vi "niDTS WLAN INSTR TX Configure Trigger.vi"(8 "error in (no error)":errorcluster, 11 "niDTS WLAN INSTR TX in":refnum<class "niDTS WLAN INSTR TX.lvclass">) -> (0 "error out":errorcluster, 3 "niDTS WLAN INSTR TX out":refnum<class "niDTS WLAN INSTR TX.lvclass">)   [LabVIEW 2015, in "niDTS WLAN.lvlib" / "niDTS WLAN INSTR TX.lvclass"]
doc: "Sets:\n\n* TriggerThreshold\n* Trigger Source\n* MinQuietTimeDuration\n* TriggerTimeout"
uses:
  niDTS WLAN INSTR TX.lvclass
  niDTS WLAN INSTR TX.lvclass/niDTS WLAN INSTR TX.ctl
  RiviInstDriver/niRfsaWlan/Objects/niRfsaWlan.lvclass
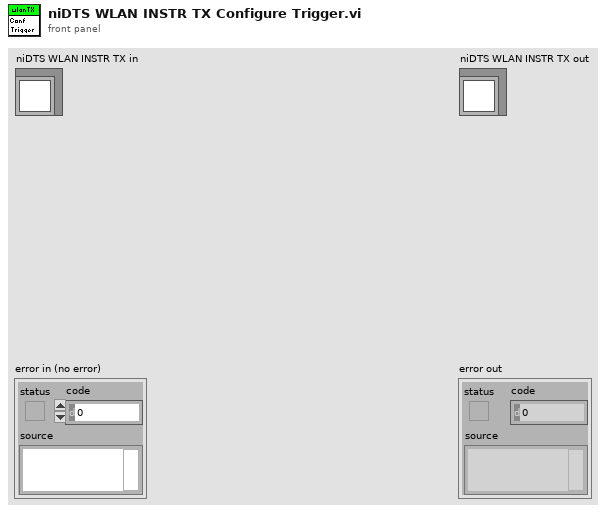
[diagram p1: front panel]
types:
  T1 = typedef "niRfsaWlan.lvclass/niRfsaWlan INC Handle.ctl" = refnum<data-value>
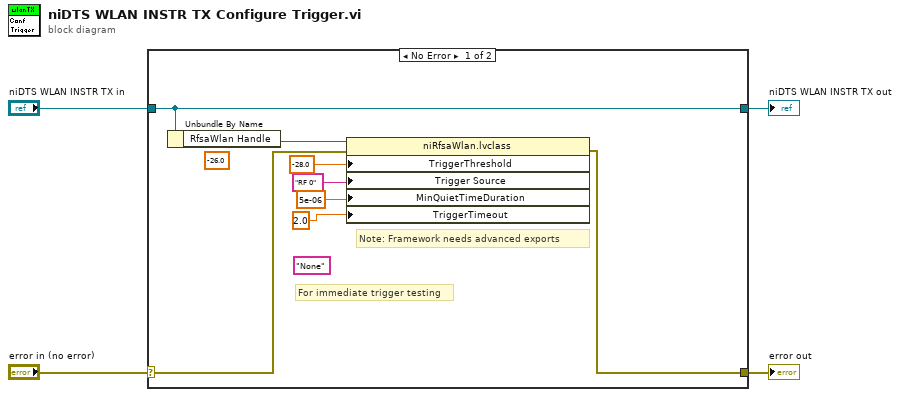
[diagram p0: block diagram]
diagram:
  n1 = case shown="No Error" "error in (no error)" {
    selector: "error in (no error)" -> [w8 w14]
    tunnel: [w7 w14] -> w3
    tunnel: [w10 w13] -> w1
    tunnel: "niDTS WLAN INSTR TX in" -> [w10 w13]
    frame No Error {
      (unwired) "None" ("Trigger Source")
      (unwired) -26.0 ("TriggerThreshold")
      # "For immediate trigger testing"
      # "Note: Framework needs advanced exports"
      n2 = Unbundle By Name(w10) -> ("RfsaWlan Handle"=w9:T1)
      n3 = property class="niRfsaWlan.lvclass"(reference=w9, error in=w8, "TriggerThreshold"=-28.0, "Trigger Source"="RF 0", "MinQuietTimeDuration"=5e-06, "TriggerTimeout"=2.0) -> (error out=w7:errorcluster)  [unwired: 1 out]
    }
    frame Error {
    }
  }
  "error out" <- w3
  "niDTS WLAN INSTR TX out" <- w1
